vi "BAM Generation Connections List.vi"(7 "State":T2=enum."Update", 8 "error in (no error)":errorcluster, 9 "index":i32, 10 "Connection Cluster":T3 {"Packets"."Identifier" format="%08x"}, 11 "BAM Gen":T1) -> (0 "error out":errorcluster, 1 "Connections":T3[](array[typedef]) {"Packets"."Identifier" format="%08x"}, 2 "Connection Cluster Out":T3 {"Packets"."Identifier" format="%08x"}, 3 "BAM Gen out":T1)   [LabVIEW 2015, in "J1939 Addon Engine.lvlib"]
uses:
  Engine/J1939 Addon Engine.lvlib
  Types/BAM Generation Connection Cluster.ctl
  J1939 Utilities/Types/CAN Outgoing Message Cluster.ctl
  Types/TP Connections List State.ctl
  Types/BAM Generation Connections List_Ref.ctl
  J1939 Utilities/J1939 Utilities.lvlib
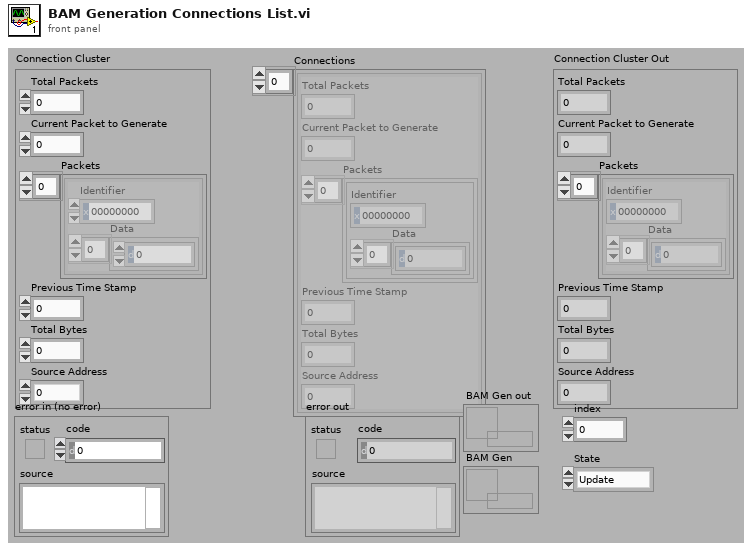
[diagram p1: front panel]
types:
  T1 = typedef "J1939 Addon Engine.lvlib/BAM Generation Connections List_Ref.ctl" = refnum<data-value>
  T2 = typedef "J1939 Addon Engine.lvlib/TP Connections List State.ctl" = enum16{"Add", "Update", "Get", "Remove", "Initialize"}
  T3 = typedef "J1939 Addon Engine.lvlib/BAM Generation Connection Cluster.ctl" = cluster{"Total Packets":u8, "Current Packet to Generate":u8, "Packets":T4[], "Previous Time Stamp":u32, "Total Bytes":u16, "Source Address":u8}
  T4 = typedef "J1939 Addon Shared.lvlib/J1939 Utilities.lvlib/CAN Outgoing Message Cluster.ctl" = cluster{"Identifier":u32, "Data":u8[]}
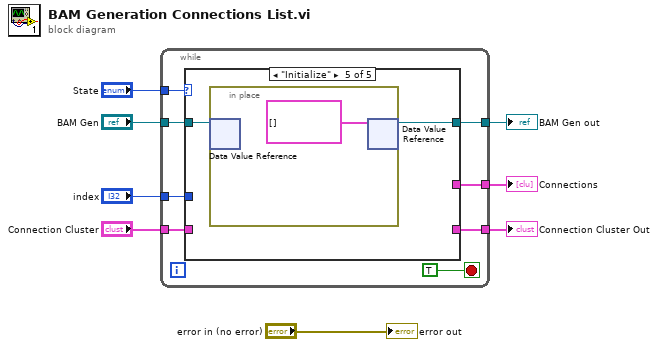
[diagram p0: block diagram]
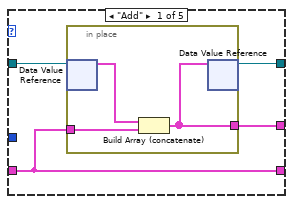
[diagram p2: hidden frame]
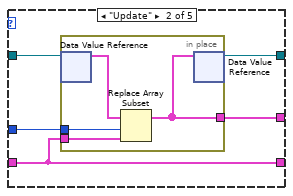
[diagram p3: hidden frame]
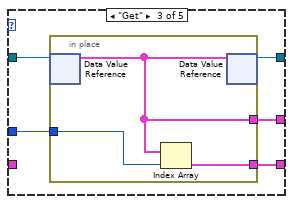
[diagram p4: hidden frame]
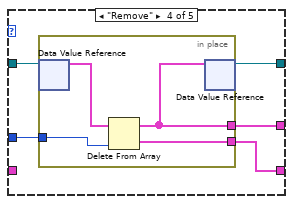
[diagram p5: hidden frame]
diagram:
  n1 = while {
    tunnel: "State" -> [w16]
    tunnel: "Connection Cluster" -> [w15]
    tunnel: "index" -> [w14]
    tunnel: [w13] -> w5
    tunnel: "BAM Gen" -> [w11]
    tunnel: [w10] -> w2
    tunnel: [w9] -> w1
    stop <- TRUE stop-if-true
    n2 = case shown="\"Initialize\"" w16 {
      tunnel: w15 -> [w19 w27 _ _ _]
      tunnel: [w20 w26 w33 w44 _] -> w9
      tunnel: w14 -> [_ w28 w37 w45 _]
      tunnel: [w19 w27 w36 w43 _] -> w13
      tunnel: w11 -> [w18 w25 w35 w42 w51]
      tunnel: [w17 w24 w34 w41 w50] -> w10
      frame "Add" {
        n3 = in-place {
          in-place-border: [w21] -> w20
          in-place-border: w19 -> [w23]
          n4 = in-place-dvr #1(w18) -> (w22:T3[])  [unwired: 1 out]
          n5 = Build Array (concatenate)(w22, w23) -> (w21:T3[])
          n6 = in-place-dvr #1(w21) -> (w17:T1)  [unwired: 1 out]
        }
      }
      frame "Update" {
        n7 = in-place {
          in-place-border: w28 -> [w32]
          in-place-border: w27 -> [w31]
          in-place-border: [w29] -> w26
          n8 = in-place-dvr #2(w25) -> (w30:T3[])  [unwired: 1 out]
          n9 = Replace Array Subset(array=w30, new element=w31, index=w32) -> (w29:T3[])
          n10 = in-place-dvr #2(w29) -> (w24:T1)  [unwired: 1 out]
        }
      }
      frame "Get" {
        n11 = in-place {
          in-place-border: w37 -> [w40]
          in-place-border: [w39] -> w36
          in-place-border: [w38] -> w33
          n12 = in-place-dvr #3(w35) -> (w38:T3[])  [unwired: 1 out]
          n13 = Index Array(array=w38, index=w40) -> (element=w39:T3)
          n14 = in-place-dvr #3(w38) -> (w34:T1)  [unwired: 1 out]
        }
      }
      frame "Remove" {
        n15 = in-place {
          in-place-border: w45 -> [w49]
          in-place-border: [w46] -> w44
          in-place-border: [w48] -> w43
          n16 = in-place-dvr #4(w42) -> (w47:T3[])  [unwired: 1 out]
          n17 = Delete From Array(array=w47, index=w49) -> (deleted portion=w48:T3, array with subset deleted=w46:T3[])  [unwired: 1 in]
          n18 = in-place-dvr #4(w46) -> (w41:T1)  [unwired: 1 out]
        }
      }
      frame "Initialize" {
        n19 = in-place {
          n20 = in-place-dvr #5(w51) -> ()  [unwired: 2 out]
          n21 = in-place-dvr #5(T3[] [] ("Connections")) -> (w50:T1)  [unwired: 1 out]
        }
      }
    }
  }
  "Connection Cluster Out" <- w5
  "Connections" <- w1
  "BAM Gen out" <- w2
  "error out" <- "error in (no error)"
